vi "Pump Off.vi"(8 "error in":errorcluster, 11 "CPC in":refnum<class "CPC.lvclass">) -> (0 "error out":errorcluster, 2 "cmdGood":bool, 3 "CPC out":refnum<class "CPC.lvclass">)   [LabVIEW 2012, in "CPC.lvclass"]
uses:
  CPC.lvclass
  Controls/CmdStruct.ctl
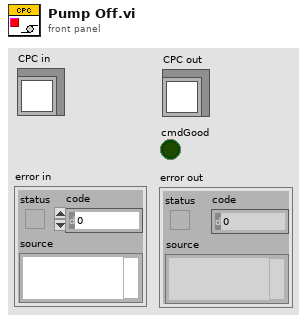
[diagram p1: front panel]
types:
  T1 = typedef "CmdStruct.ctl" = cluster{"Cmd":u8, "x":i64, "y":i64, "Display":string}
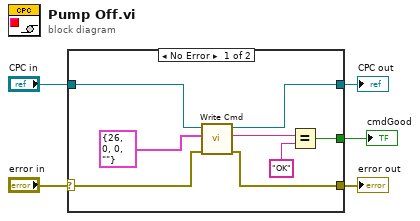
[diagram p0: block diagram]
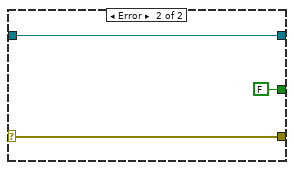
[diagram p2: hidden frame]
diagram:
  n1 = case shown="No Error" "error in" {
    selector: "error in" -> [w11 w16]
    tunnel: [w10 w16] -> w4
    tunnel: [w12 w15] -> w2
    tunnel: "CPC in" -> [w13 w15]
    tunnel: [w6 FALSE] -> w1
    frame No Error {
      n2 = call-dynamic "Write Cmd.vi"("error in"=w11, "CmdStruct"=T1 {"Cmd"=26, "x"=0, "y"=0, "Display"=""}, "CPC in"=w13) -> ("error out"=w10:errorcluster, "Buffer"=w8:string, "CPC out"=w12:refnum<class "CPC.lvclass">)  [unwired: 6 in]
      n3 = Equal?(x=w8, y="OK") -> (x = y?=w6:bool)
    }
    frame Error {
    }
  }
  "error out" <- w4
  "CPC out" <- w2
  "cmdGood" <- w1
